vi "Config Offset.vi"(11 "Offset":sgl[][](array[numeric]) caption="OFFSET") -> (3 "Offset Out":sgl[][](array[numeric]) caption="OFFSET")   [LabVIEW 2014, in "CAP-USB-1.lvlib" / "CAP-USB-1.lvclass"]
doc: "Pantalla de configuracion de offset de transductores"
uses:
  CAP-USB-1Class/CAP-USB-1.lvclass
panel:
  in  "Cancelar":bool
  in  "Aceptar":bool
  # "1-16"
  # "17-32"
  # "33-48"
  # "49-64"
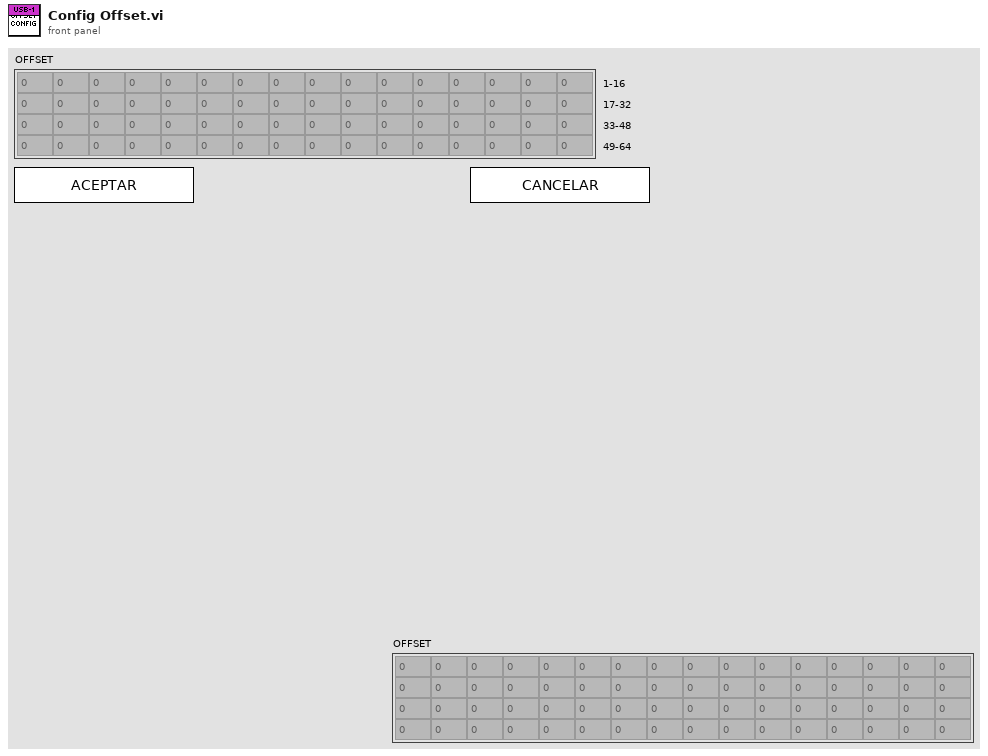
[diagram p1: front panel]
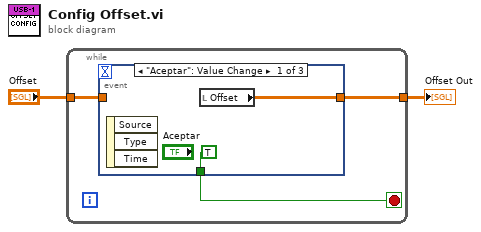
[diagram p0: block diagram]
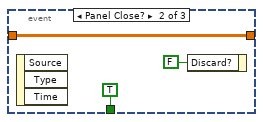
[diagram p2: hidden frame]
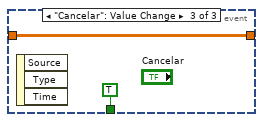
[diagram p3: hidden frame]
diagram:
  n1 = while {
    tunnel: "Offset" -> [w4]
    tunnel: [w3] -> w1
    stop <- w5 stop-if-true
    n2 = event shown="[0] \"Aceptar\": Value Change" {
      selector: _ -> [_ _ _]
      dyn-events: _ -> [_ _ _]
      timeout: _ -> [_ _ _]
      tunnel: [TRUE ("Config") TRUE ("Config") TRUE ("Config")] -> w5
      tunnel: w4 -> [_ w10 w12]
      tunnel: [w7 w10 w12] -> w3
      event "Aceptar": Value Change {
        n3 = event-data() -> ()  [unwired: 1 in, 3 out]
        n4 = local read "Offset"() -> (w7:sgl[][])
      }
      event Panel Close? {
        n5 = event-data() -> ()  [unwired: 1 in, 3 out]
        n6 = event-data("Discard?"=FALSE) -> ()  [unwired: 1 in, 1 out]
      }
      event "Cancelar": Value Change {
        n7 = event-data() -> ()  [unwired: 1 in, 3 out]
      }
    }
  }
  "Offset Out" <- w1
